vi "Set Dialog Properties.vi"(8 "error in (no error)":errorcluster, 10 "Boolean":bool, 11 "VI in":refnum<vi>) -> (0 "error out":errorcluster, 3 "VI out":refnum<vi>)   [LabVIEW 2017]
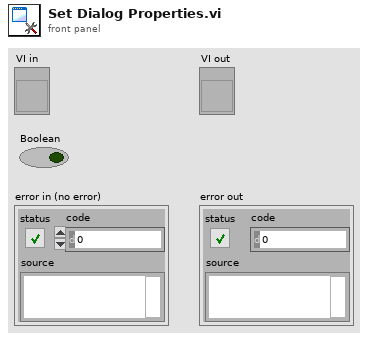
[diagram p1: front panel]
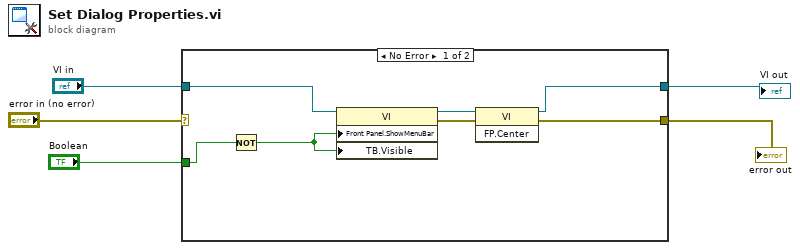
[diagram p0: block diagram]
diagram:
  n1 = case shown="No Error" "error in (no error)" {
    selector: "error in (no error)" -> [_ w13]
    tunnel: [w8 w13] -> w5
    tunnel: [w9 w14] -> w4
    tunnel: "Boolean" -> [w7 _]
    tunnel: "VI in" -> [w12 w14]
    frame No Error {
      n2 = Not(x=w7) -> (.not. x?=w6:bool)
      n3 = property class="VI"(reference=w12, "Front Panel.ShowMenuBar"=w6, "TB.Visible"=w6) -> (reference out=w11:refnum<vi>, error out=w10:errorcluster)  [unwired: 1 in]
      n4 = invoke class="VI" method="FP.Center"(reference=w11, error in=w10) -> (reference out=w9:refnum<vi>, error out=w8:errorcluster)  [unwired: 1 in, 1 out]
    }
    frame Error {
    }
  }
  "error out" <- w5
  "VI out" <- w4
